vi "CameraAttributeSearch.vi"() -> ()   [LabVIEW 2022 SP3]
uses:
  <vilib>/userdefined/High Color/IMAQdx.ctl
  <vilib>/vision/driver/IMAQdx.llb/IMAQdx Attribute Type.ctl
  <vilib>/regexp/Match Regular Expression.xnode
  <vilib>/vision/driver/NI_Vision_Acquisition_Software.lvlib
  <resource>/objmgr/imaqdx.rc
panel:
  out "ValueBool":bool
  out "EnumStrings[]":string[](array[string])
  out "ValueString":string
  out "ValueDBL":dbl
  out "ValueI64":i64
  out "ValueU32":u32
  out "Ready":bool=TRUE
  out "Attributes":T2(array[cluster])
  in  "Attribute search":string
  in  "stop":bool
  in  "Session In":T3="16511205"
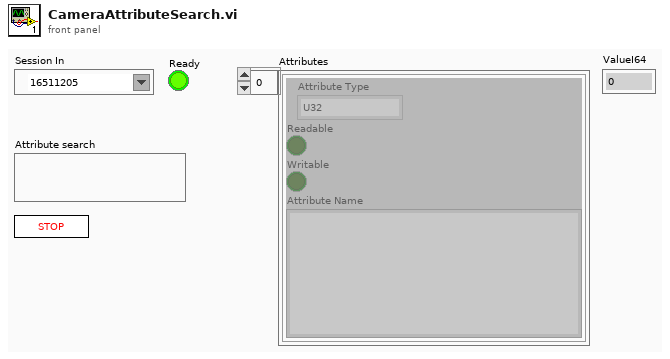
[diagram p1: front panel]
types:
  T1 = typedef "NI_Vision_Acquisition_Software.lvlib/IMAQdx Attribute Type.ctl" = enum32{"U32", "I64", "DBL", "String", "Enum", "Bool", "Command"}
  T2 = cluster{"Attribute Type":T1, "Readable":bool, "Writable":bool, "Attribute Name":string}[]
  T3 = typedef "IMAQdx.ctl" = refnum<k21>
  T4 = cluster{"Attribute Type":T1, "Readable":bool, "Writable":bool, "Attribute Name":string}
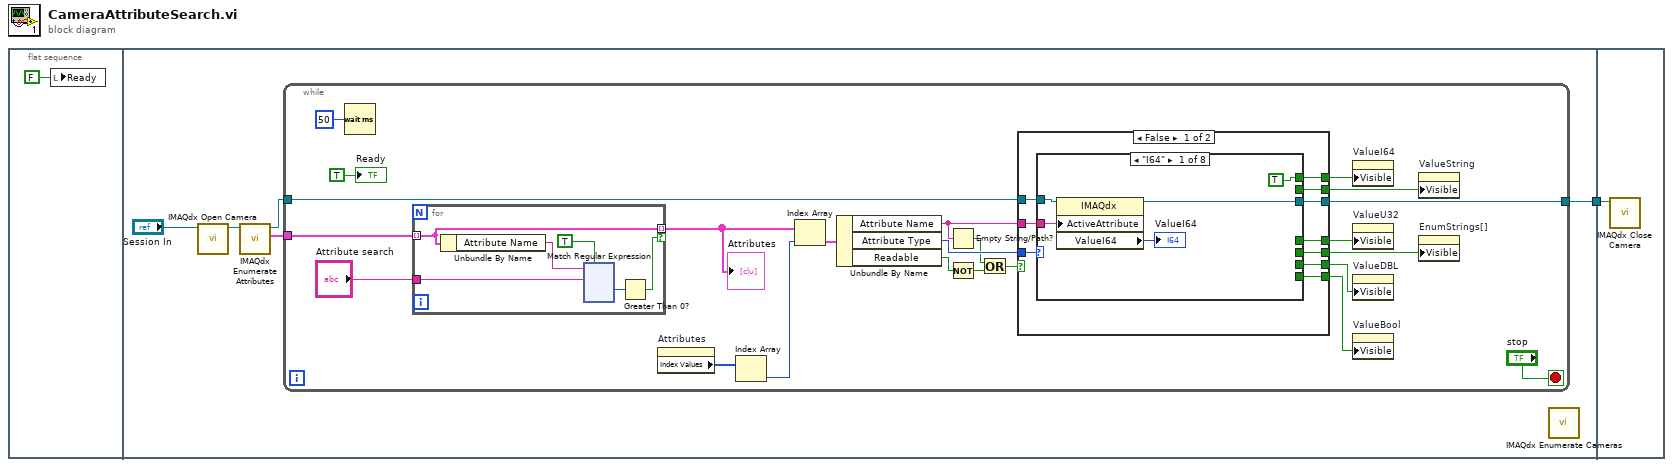
[diagram p0: block diagram]
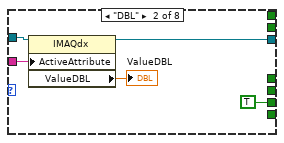
[diagram p2: hidden frame]
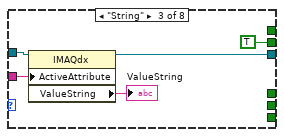
[diagram p3: hidden frame]
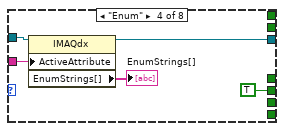
[diagram p4: hidden frame]
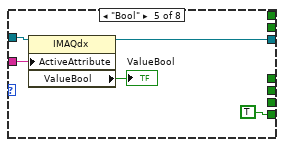
[diagram p5: hidden frame]
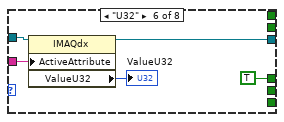
[diagram p6: hidden frame]
diagram:
  n1 = flat-sequence {
    tunnel: [w3] -> w1
    tunnel: w1 -> [w197]
    frame #0 {
      n2 = local write "Ready"(FALSE) -> ()
    }
    frame #1 {
      n3 = call <vilib>:"IMAQdx Open Camera.vi"("Session In"="Session In") -> ("Session Out"=w7:T3)  [unwired: 9 in, 1 out]
      n4 = call <vilib>:"IMAQdx Enumerate Attributes.vi"("Session In"=w7) -> ("Attribute Information Array"=w6:T2, "Session Out"=w4:T3)  [unwired: 8 in, 1 out]
      n5 = while {
        tunnel: w6 -> [w28]
        tunnel: w4 -> [w25]
        tunnel: [w24] -> w3
        stop <- "stop" stop-if-true
        n6 = Wait (ms)(milliseconds to wait=u32 50) -> ()  [unwired: 1 out]
        n7 = for {
          tunnel: w28 -> [w78] mode=indexing
          tunnel: "Attribute search" -> [w79]
          tunnel: [w78] -> w22 mode=indexing if=w75
          n8 = Unbundle By Name(w78) -> ("Attribute Name"=w77:string)
          n9 = xnode "Match Regular Expression"("input string"=w77, "regular expression"=w79, "ignore case? (F)"=TRUE) -> ("offset past match"=w76:i32)  [unwired: 3 in, 4 out]
          n10 = Greater Than 0?(x=w76) -> (x > 0?=w75:bool)
        }
        "Attributes" <- w22
        n11 = property on="Attributes" class="Arr (strict)"() -> ("Index Values"=w21:u32[])  [unwired: 2 in, 2 out]
        n12 = Index Array(array=w21) -> (element=w20:u32)  [unwired: 1 in]
        n13 = Index Array(array=w22, index=w20) -> (element=w19:T4)
        n14 = Unbundle By Name(w19) -> ("Attribute Name"=w18:string, "Attribute Type"=w23:T1, "Readable"=w10:bool)
        n15 = Empty String/Path?(string/path=w18) -> (empty?=w17:bool)
        n16 = Not(x=w10) -> (.not. x?=w8:bool)
        n17 = Or(x=w17, y=w8) -> (x .or. y?=w9:bool)
        n18 = case shown="False" w9 {
          tunnel: w25 -> [w40 w73]
          tunnel: [w39 w73] -> w24
          tunnel: w23 -> [w38 _]
          tunnel: w18 -> [w37 _]
          tunnel: [w36 _] -> w16
          tunnel: [w35 _] -> w15
          tunnel: [w34 _] -> w14
          tunnel: [w33 _] -> w13
          tunnel: [w32 _] -> w12
          tunnel: [w31 _] -> w11
          frame False {
            n19 = case shown="\"I64\"" w38 {
              tunnel: w40 -> [w45 w50 w55 w60 w65 w70 w71 w72]
              tunnel: [w44 w49 w54 w59 w64 w69 w71 w72] -> w39
              tunnel: w37 -> [w43 w48 w53 w58 w63 w68 _ _]
              tunnel: [TRUE _ _ _ _ _ _ _] -> w36
              tunnel: [_ TRUE _ _ _ _ _ _] -> w35
              tunnel: [_ _ TRUE _ _ _ _ _] -> w34
              tunnel: [_ _ _ TRUE _ _ _ _] -> w33
              tunnel: [_ _ _ _ TRUE _ _ _] -> w32
              tunnel: [_ _ _ _ _ TRUE _ _] -> w31
              frame "I64" {
                n20 = property class="IMAQdx"(reference=w45, "ActiveAttribute"=w43) -> (reference out=w44:T3, "ValueI64"=→"ValueI64":i64)  [unwired: 1 in, 1 out]
              }
              frame "DBL" {
                n21 = property class="IMAQdx"(reference=w50, "ActiveAttribute"=w48) -> (reference out=w49:T3, "ValueDBL"=→"ValueDBL":dbl)  [unwired: 1 in, 1 out]
              }
              frame "String" {
                n22 = property class="IMAQdx"(reference=w55, "ActiveAttribute"=w53) -> (reference out=w54:T3, "ValueString"=→"ValueString":string)  [unwired: 1 in, 1 out]
              }
              frame "Enum" {
                n23 = property class="IMAQdx"(reference=w60, "ActiveAttribute"=w58) -> (reference out=w59:T3, "EnumStrings[]"=→"EnumStrings[]":string[])  [unwired: 1 in, 1 out]
              }
              frame "Bool" {
                n24 = property class="IMAQdx"(reference=w65, "ActiveAttribute"=w63) -> (reference out=w64:T3, "ValueBool"=→"ValueBool":bool)  [unwired: 1 in, 1 out]
              }
              frame "U32" {
                n25 = property class="IMAQdx"(reference=w70, "ActiveAttribute"=w68) -> (reference out=w69:T3, "ValueU32"=→"ValueU32":u32)  [unwired: 1 in, 1 out]
              }
              frame "Command" {
              }
              frame Default {
              }
            }
          }
          frame True {
          }
        }
        n26 = property on="ValueI64" class="DigNum (strict)"("Visible"=w16) -> ()  [unwired: 2 in, 2 out]
        n27 = property on="ValueU32" class="DigNum (strict)"("Visible"=w11) -> ()  [unwired: 2 in, 2 out]
        n28 = property on="ValueDBL" class="DigNum (strict)"("Visible"=w15) -> ()  [unwired: 2 in, 2 out]
        n29 = property on="ValueBool" class="Bool (strict)"("Visible"=w12) -> ()  [unwired: 2 in, 2 out]
        n30 = property on="ValueString" class="Str"("Visible"=w14) -> ()  [unwired: 2 in, 2 out]
        n31 = property on="EnumStrings[]" class="Arr (strict)"("Visible"=w13) -> ()  [unwired: 2 in, 2 out]
        "Ready" <- TRUE
      }
      n32 = call <vilib>:"IMAQdx Enumerate Cameras.vi"() -> ()  [unwired: 10 in, 2 out]
    }
    frame #2 {
      n33 = call <vilib>:"IMAQdx Close Camera.vi"("Session In"=w197) -> ()  [unwired: 10 in, 1 out]
    }
  }
